vi "LaserFinding_Lines_v3.vi"(0 "Image In":T2, 7 "error in":errorcluster) -> (20 "Image Out":T2, 21 "Straight Edge (Find Vert. Edge)":T1 {"Point2 (Real-World)"."Y" format="%.2f"; "Point2 (Real-World)"."X" format="%.2f"; "Point1 (Real-World)"."Y" format="%.2f"; "Point1 (Real-World)"."X" format="%.2f"; "Point2 (Pixels)"."Y" format="%.2f"; "Point2 (Pixels)"."X" format="%.2f"; "Point1 (Pixels)"."Y" format="%.2f"; "Point1 (Pixels)"."X" format="%.2f"}, 22 "Straight Edge (Find Horiz. Edge)":T1 {"Point2 (Real-World)"."Y" format="%.2f"; "Point2 (Real-World)"."X" format="%.2f"; "Point1 (Real-World)"."Y" format="%.2f"; "Point1 (Real-World)"."X" format="%.2f"; "Point2 (Pixels)"."Y" format="%.2f"; "Point2 (Pixels)"."X" format="%.2f"; "Point1 (Pixels)"."Y" format="%.2f"; "Point1 (Pixels)"."X" format="%.2f"}, 27 "error out":errorcluster)   [LabVIEW 2014]
uses:
  <vilib>/vision/Image Controls.llb/IMAQ Image.ctl
  <vilib>/vision/Measure.llb/Straight Edge Options.ctl
  <vilib>/vision/Measure.llb/Straight Edge Process.ctl
  <vilib>/vision/Measure.llb/Edge Options.ctl
  <vilib>/vision/Measure.llb/Edge Polarity.ctl
  <vilib>/vision/NI_Vision_Development_Module.lvlib
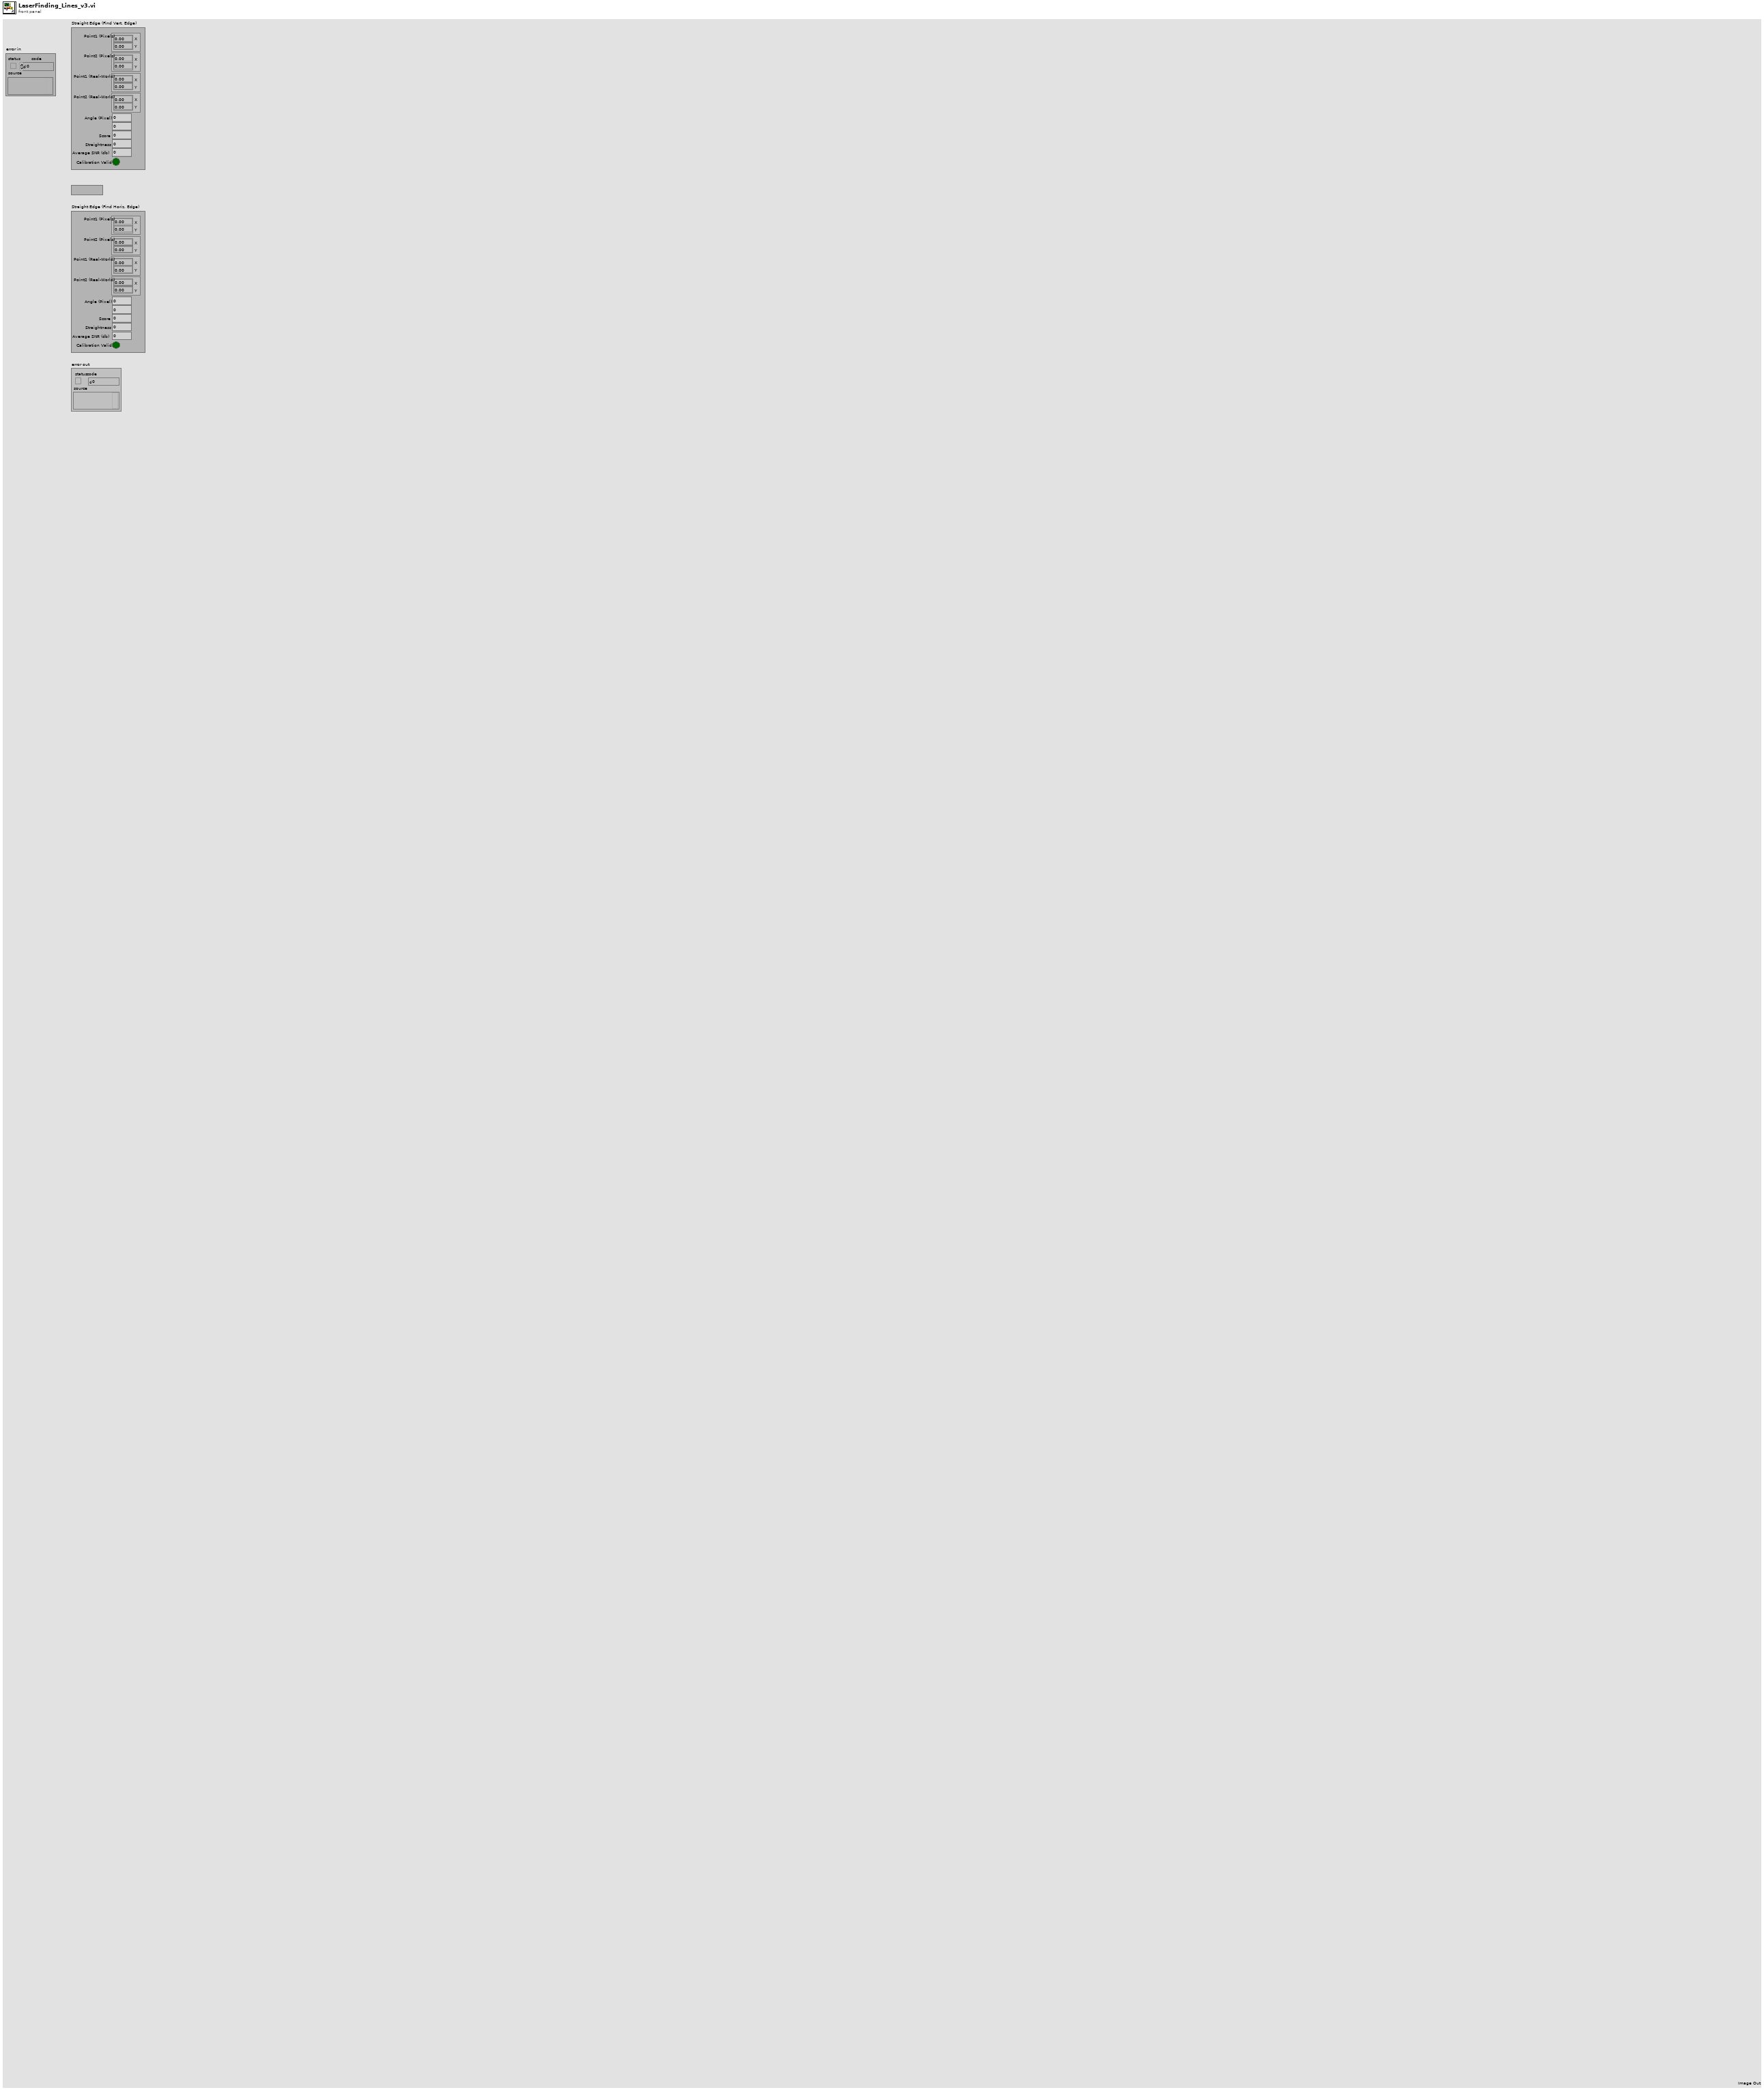
[diagram p1: front panel]
types:
  T1 = cluster{"Point1 (Pixels)":cluster{"X":sgl, "Y":sgl}, "Point2 (Pixels)":cluster{"X":sgl, "Y":sgl}, "Point1 (Real-World)":cluster{"X":sgl, "Y":sgl}, "Point2 (Real-World)":cluster{"X":sgl, "Y":sgl}, "Angle (Pixel)":dbl, "Angle (Real-World)":dbl, "Score":dbl, "Straightness":dbl, "Average SNR (db)":dbl, "Calibration Valid":bool}
  T2 = typedef "IMAQ Image.ctl" = refnum<image>
  T3 = typedef "Edge Options.ctl" = cluster{"Edge Polarity":T4, "Kernel Size":u32, "Width":u32, "Minimum Edge Strength":sgl, "Interpolation Type":enum32{"Zero Order", "Bilinear", "Quadratic", "Cubic", "Bilinear Fixed"}, "Data Processing Method":enum32{"Average", "Median"}}
  T4 = typedef "Edge Polarity.ctl" = u32
  T5 = cluster{"Search Direction":u32, "Edge Options":T3, "Show Search Area":bool, "Show Search Lines":bool, "Show Edges Found":bool, "Show Result":bool, "Search Area Color":u32, "Search Lines Color":u32, "Edge Locations Color":u32, "Result Color":u32, "Overlay Group Name":string}
  T6 = typedef "Straight Edge Options.ctl" = cluster{"Number of Lines":i32, "Type":T7, "Min. Score":dbl, "Max. Score":dbl, "Orientation":dbl, "Angle Range":dbl, "Angle Tolerance":dbl, "Step Size":u32, "Min. SNR (db)":dbl, "Min. Points (%)":dbl, "Hough Iterations":i32}
  T7 = typedef "Straight Edge Process.ctl" = enum32{"First Edge Rake", "Best Edge Rake", "Hough Edge Rake", "First Edge Projection", "Best Edge Projection"}
  T8 = cluster{"Global Rectangle":i32[], "Contours":cluster{"ID":enum32{"External", "Internal"}, "Type":u32, "Coordinates":i32[]}[]}
  T9 = cluster{"Brightness":sgl, "Contrast":sgl, "Gamma":sgl}
  T10 = typedef "Image Type" = u32
  T11 = cluster{"Point1 (Pixels)":cluster{"X":sgl, "Y":sgl}, "Point2 (Pixels)":cluster{"X":sgl, "Y":sgl}, "Point1 (Real-World)":cluster{"X":sgl, "Y":sgl}, "Point2 (Real-World)":cluster{"X":sgl, "Y":sgl}, "Angle (Pixel)":dbl, "Angle (Real-World)":dbl, "Score":dbl, "Straightness":dbl, "Average SNR (db)":dbl, "Calibration Valid":bool}[]
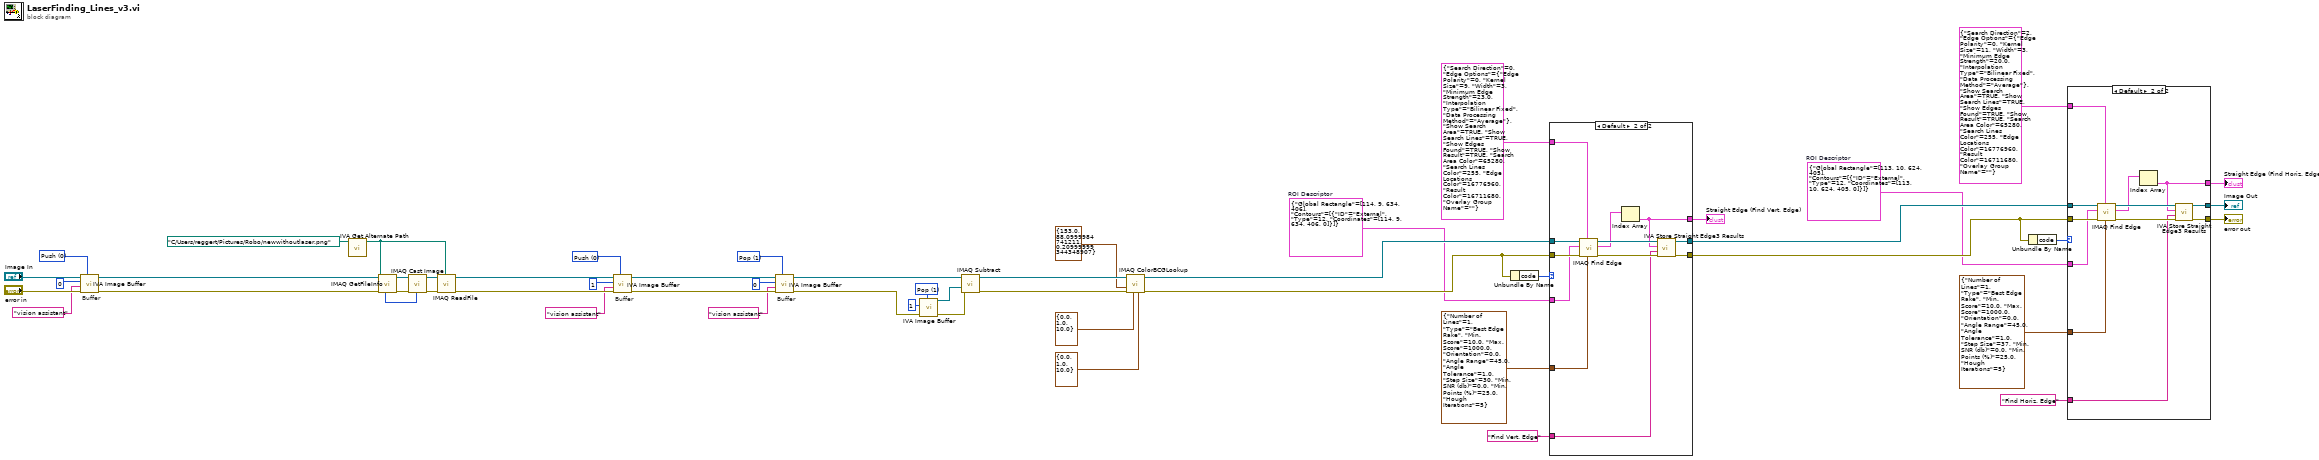
[diagram p0: block diagram]
diagram:
  w8 = T8 {"Global Rectangle"=[113, 10, 624, 405], "Contours"=[{"ID"=enum."External", "Type"=12, "Coordinates"=[113, 10, 624, 405, 0]}]}  # ROI Descriptor
  w16 = T8 {"Global Rectangle"=[114, 9, 634, 406], "Contours"=[{"ID"=enum."External", "Type"=12, "Coordinates"=[114, 9, 634, 406, 0]}]}  # ROI Descriptor
  w28 = u16 1 items=["Push", "Pop", "Reset"] ("Function")
  w31 = u16 1 items=["Push", "Pop", "Reset"] ("Function")
  w36 = u16 0 items=["Push", "Pop", "Reset"] ("Function")
  w49 = u16 0 items=["Push", "Pop", "Reset"] ("Function")
  # "Buffer"
  # "Buffer"
  # "Buffer"
  n1 = call <vilib>:"IVA Image Buffer.vi"("Function"=w49, "error in (no error)"="error in", "Prefix"="vision assistant", "Buffer #"=0, "Image In"="Image In") -> ("error out"=w50:errorcluster, "Image Out"=w43:T2)  [unwired: 5 out]
  n2 = call <vilib>:"IVA Get Alternate Path.vi"("Path In"=path "C:/Users/reggert/Pictures/Robo/newwithoutlaser.png" ("File Path")) -> ("Path Out"=w39:path)  [unwired: 10 out]
  n3 = call "IMAQ GetFileInfo"("error in (no error)"=w50, "File Path"=w39) -> ("error out"=w45:errorcluster, "Image Type"=w41:T10)  [unwired: 8 out]
  n4 = call "IMAQ Cast Image"("Image Type"=w41, "error in (no error)"=w45, "Image Src"=w43) -> ("error out"=w44:errorcluster, "Image Dst Out"=w42:T2)  [unwired: 3 in, 4 out]
  n5 = call "IMAQ ReadFile"("File Path"=w39, "error in (no error)"=w44, "Image"=w42) -> ("error out"=w46:errorcluster, "Image Out"=w38:T2)  [unwired: 2 in, 5 out]
  n6 = call <vilib>:"IVA Image Buffer.vi"("Function"=w36, "error in (no error)"=w46, "Prefix"="vision assistant", "Buffer #"=1, "Image In"=w38) -> ("error out"=w37:errorcluster, "Image Out"=w33:T2)  [unwired: 5 out]
  n7 = call <vilib>:"IVA Image Buffer.vi"("Function"=w31, "error in (no error)"=w37, "Prefix"="vision assistant", "Buffer #"=0, "Image In"=w33) -> ("error out"=w32:errorcluster, "Image Out"=w24:T2)  [unwired: 5 out]
  n8 = call <vilib>:"IVA Image Buffer.vi"("Function"=w28, "error in (no error)"=w32, "Buffer #"=1) -> ("error out"=w25:errorcluster, "Image Out"=w26:T2)  [unwired: 2 in, 5 out]
  n9 = call "IMAQ Subtract"("Image Src A"=w24, "Image Src B"=w26, "error in (no error)"=w25) -> ("Image Dst Out"=w22:T2, "error out"=w23:errorcluster)  [unwired: 2 in, 2 out]
  n10 = call "IMAQ ColorBCGLookup"("Blue BCG Values"=T9 {"Brightness"=0.0, "Contrast"=1.0, "Gamma"=10.0}, "Green BCG Values"=T9 {"Brightness"=0.0, "Contrast"=1.0, "Gamma"=10.0}, "error in (no error)"=w23, "Red BCG Values"=T9 {"Brightness"=153.0, "Contrast"=88.1, "Gamma"=0.21}, "Image Src"=w22) -> ("error out"=w21:errorcluster, "Image Dst Out"=w17:T2)  [unwired: 2 in, 3 out]
  n11 = Unbundle By Name(w21) -> ("code"=w13:i32)
  n12 = case shown="Default" w13 {
    tunnel: w17 -> [w53 w65]
    tunnel: w21 -> [_ w64]
    tunnel: w16 -> [_ w58]
    tunnel: [w53 w62] -> w9
    tunnel: [_ w60] -> w15
    tunnel: "Find Vert. Edge" ("Step Name") -> [_ w59]
    tunnel: T6 {"Number of Lines"=1, "Type"=enum."Best Edge Rake", "Min. Score"=10.0, "Max. Score"=1000.0, "Orientation"=0.0, "Angle Range"=45.0, "Angle Tolerance"=1.0, "Step Size"=30, "Min. SNR (db)"=0.0, "Min. Points (%)"=25.0, "Hough Iterations"=5} ("Fit Options") -> [_ w57]
    tunnel: T5 {"Search Direction"=0, "Edge Options"={"Edge Polarity"=0, "Kernel Size"=9, "Width"=3, "Minimum Edge Strength"=23.0, "Interpolation Type"=enum."Bilinear Fixed", "Data Processing Method"=enum."Average"}, "Show Search Area"=TRUE, "Show Search Lines"=TRUE, "Show Edges Found"=TRUE, "Show Result"=TRUE, "Search Area Color"=65280, "Search Lines Color"=255, "Edge Locations Color"=16776960, "Result Color"=16711680, "Overlay Group Name"=""} ("Options") -> [_ w56]
    tunnel: [_ w54] -> w10
    frame -1074396199, -1074396198 {
      # "Discard Coordinate System Error"
    }
    frame Default {
      n13 = call "IMAQ Find Edge"("Line Fit Options"=w57, "Options"=w56, "error in (no error)"=w64, "ROI Descriptor"=w58, "Image"=w65) -> ("error out"=w61:errorcluster, "Straight Edges"=w55:T11, "Image Out"=w63:T2)  [unwired: 1 in, 3 out]
      n14 = Index Array(array=w55) -> (element=w54:T1)  [unwired: 1 in]
      n15 = call <vilib>:"IVA Store Straight Edge3 Results.vi"("error in (no error)"=w61, "Step Name"=w59, "Straight Edge"=w54, "Image in"=w63) -> ("error out"=w60:errorcluster, "Image dup"=w62:T2)  [unwired: 1 in, 5 out]
    }
  }
  "Straight Edge (Find Vert. Edge)" <- w10
  n16 = Unbundle By Name(w15) -> ("code"=w4:i32)
  n17 = case shown="Default" w4 {
    tunnel: w9 -> [w66 w78]
    tunnel: w15 -> [_ w77]
    tunnel: w8 -> [_ w71]
    tunnel: [w66 w75] -> w7
    tunnel: [_ w73] -> w6
    tunnel: "Find Horiz. Edge" ("Step Name") -> [_ w72]
    tunnel: T6 {"Number of Lines"=1, "Type"=enum."Best Edge Rake", "Min. Score"=10.0, "Max. Score"=1000.0, "Orientation"=0.0, "Angle Range"=45.0, "Angle Tolerance"=1.0, "Step Size"=37, "Min. SNR (db)"=0.0, "Min. Points (%)"=25.0, "Hough Iterations"=5} ("Fit Options") -> [_ w70]
    tunnel: T5 {"Search Direction"=2, "Edge Options"={"Edge Polarity"=0, "Kernel Size"=11, "Width"=3, "Minimum Edge Strength"=20.0, "Interpolation Type"=enum."Bilinear Fixed", "Data Processing Method"=enum."Average"}, "Show Search Area"=TRUE, "Show Search Lines"=TRUE, "Show Edges Found"=TRUE, "Show Result"=TRUE, "Search Area Color"=65280, "Search Lines Color"=255, "Edge Locations Color"=16776960, "Result Color"=16711680, "Overlay Group Name"=""} ("Options") -> [_ w69]
    tunnel: [_ w67] -> w1
    frame -1074396199, -1074396198 {
      # "Discard Coordinate System Error"
    }
    frame Default {
      n18 = call "IMAQ Find Edge"("Line Fit Options"=w70, "Options"=w69, "error in (no error)"=w77, "ROI Descriptor"=w71, "Image"=w78) -> ("error out"=w74:errorcluster, "Straight Edges"=w68:T11, "Image Out"=w76:T2)  [unwired: 1 in, 3 out]
      n19 = Index Array(array=w68) -> (element=w67:T1)  [unwired: 1 in]
      n20 = call <vilib>:"IVA Store Straight Edge3 Results.vi"("error in (no error)"=w74, "Step Name"=w72, "Straight Edge"=w67, "Image in"=w76) -> ("error out"=w73:errorcluster, "Image dup"=w75:T2)  [unwired: 1 in, 5 out]
    }
  }
  "Image Out" <- w7
  "error out" <- w6
  "Straight Edge (Find Horiz. Edge)" <- w1
